vi "SigGenPwrMtr.vi"() -> ()   [LabVIEW 2009]
panel:
  out "Power returned (dBm)":dbl(graph)
  in  "RF Power Level (dBm)":dbl=-80.0 min=-120.0 max=20.0 step=2.0 format="%#_9g"
  in  "RF Frequency  (GHz)":dbl=2.809 min=0.6 max=3.0 step=0.001 format="%#_9g"
  out "RF Power":bool
  in  "RF ON/OFF":bool
  in  "SET FREQ":bool
  in  "SET POWER":bool
  out "Power":dbl
  out "Freq (GHz)":dbl format="%#_10e"
  in  "error in (no error)":errorcluster
  out "error out":errorcluster
  in  "STATUS":bool
  in  "STOP":bool
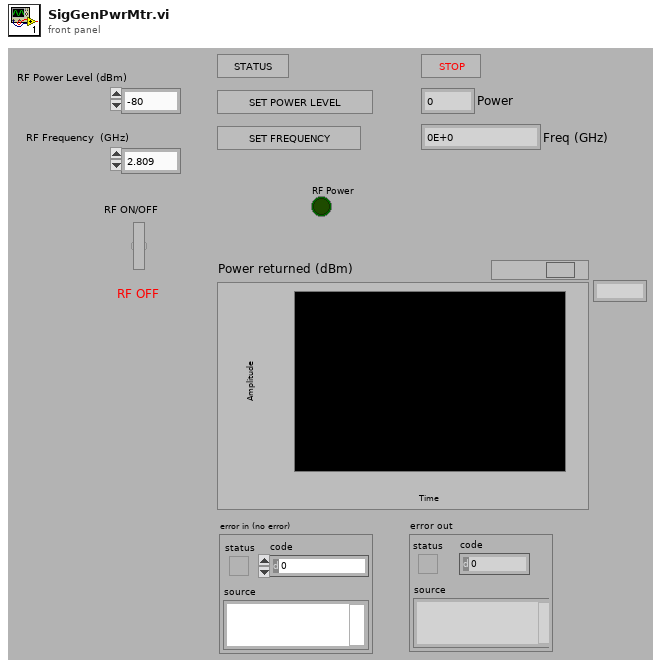
[diagram p1: front panel]
types:
  T1 = enum16{"N1911A", "Siggen", "34980a", "E4418B", "Rvp8"}
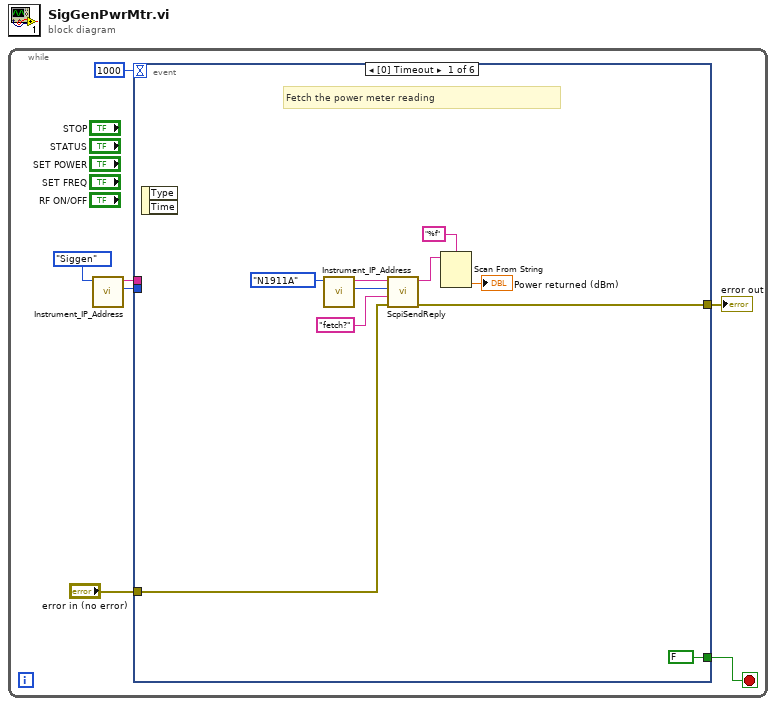
[diagram p0: block diagram]
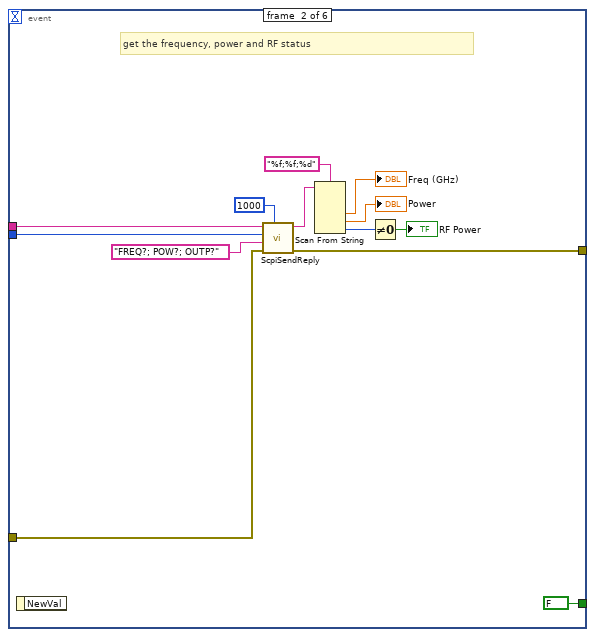
[diagram p2: hidden frame]
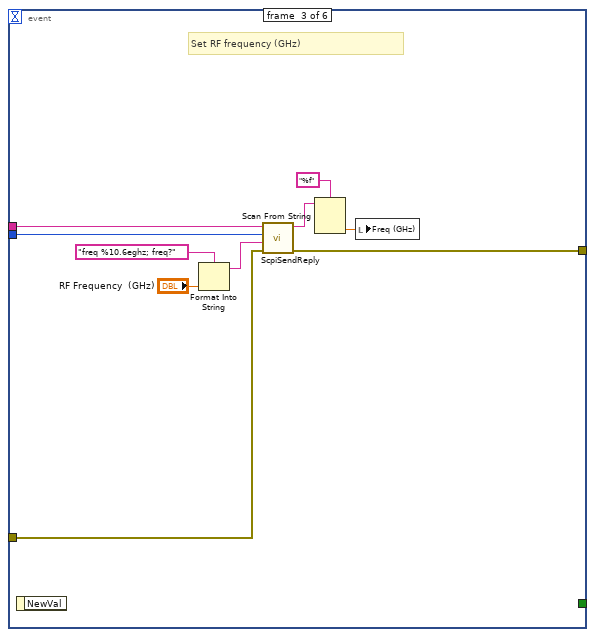
[diagram p3: hidden frame]
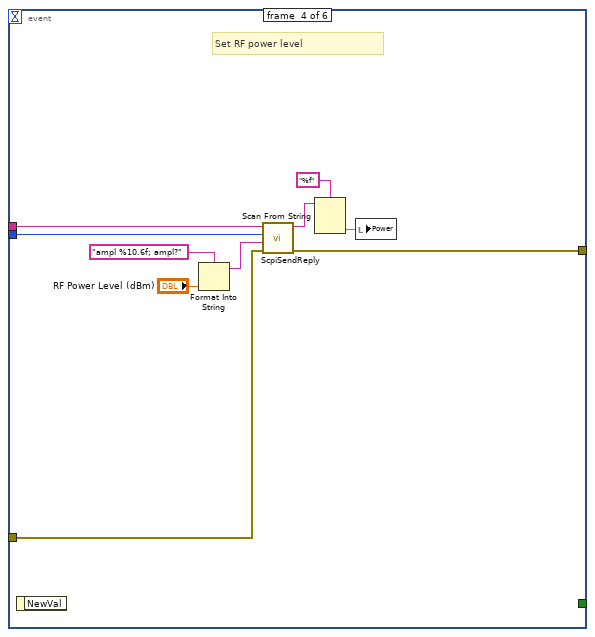
[diagram p4: hidden frame]
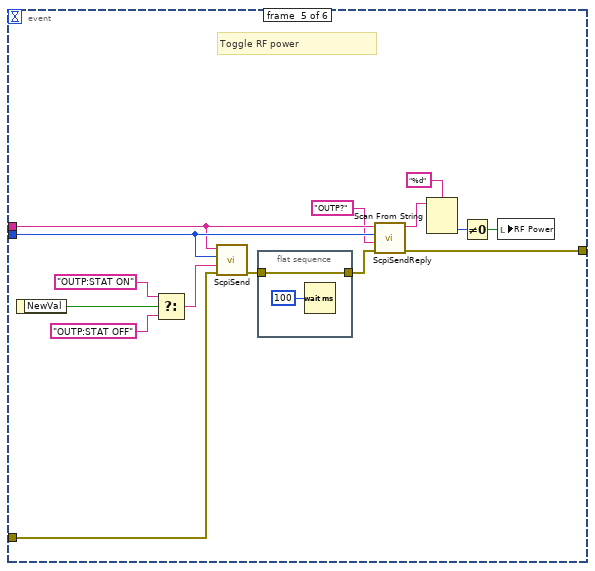
[diagram p5: hidden frame]
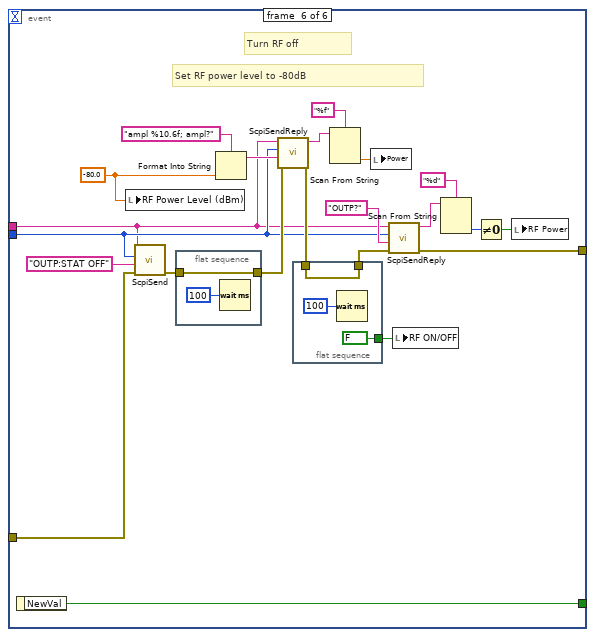
[diagram p6: hidden frame]
diagram:
  n1 = while {
    stop <- w7 stop-if-true
    n2 = call "Instrument_IP_Address.vi"("Instrument"=T1."Siggen") -> ("Port"=w1:u16, "IP Address"=w2:string)  [unwired: 9 in]
    n3 = event shown="[0] Timeout" {
      selector: _ -> [_ _ _ _ _ _]
      dyn-events: _ -> [_ _ _ _ _ _]
      timeout: 1000 -> [_ _ _ _ _ _]
      tunnel: [FALSE ("NewVal") FALSE ("NewVal") _ _ _ w89] -> w7
      tunnel: "error in (no error)" -> [w9 w28 w32 w43 w55 w83]
      tunnel: [w8 w27 w31 w42 w59 w82] -> w5
      tunnel: w2 -> [_ w19 w34 w45 w57 w70]
      tunnel: w1 -> [_ w18 w33 w44 w58 w71]
      event #0 {
        # "Fetch the power meter reading"
        n4 = event-data() -> ()  [unwired: 1 in, 2 out]
        n5 = call "Instrument_IP_Address.vi"("Instrument"=T1."N1911A") -> ("Port"=w16:u16, "IP Address"=w15:string)  [unwired: 9 in]
        n6 = call "ScpiSendReply.vi"("error in (no error)"=w9, "Command"="fetch?" ("format string"), "TCP port"=w16, "IP Address"=w15) -> ("Error out"=w8:errorcluster, "Reply"=w11:string)  [unwired: 5 in]
        n7 = Scan From String(format string="%f", input string=w11) -> (output 1=→"Power returned (dBm)":dbl)  [unwired: 3 in, 3 out]
      }
      event #1 {
        # "get the frequency, power and RF status"
        n8 = event-data() -> ()  [unwired: 1 in, 1 out]
        n9 = call "ScpiSendReply.vi"("TCP Timeout mS"=1000, "error in (no error)"=w28, "Command"="FREQ?; POW?; OUTP?" ("format string"), "TCP port"=w18, "IP Address"=w19) -> ("Error out"=w27:errorcluster, "Reply"=w25:string)  [unwired: 4 in]
        n10 = Scan From String(format string="%f;%f;%d", input string=w25) -> (output 1=→"Freq (GHz)":dbl, output 2=→"Power":dbl, output 3=w20:i32)  [unwired: 5 in, 3 out]
        n11 = Not Equal To 0?(x=w20) -> (x != 0?=→"RF Power":bool)
      }
      event #2 {
        # "Set RF frequency (GHz)"
        n12 = event-data() -> ()  [unwired: 1 in, 1 out]
        n13 = Format Into String(format string="freq %10.6eghz; freq?", "RF Frequency  (GHz)") -> (resulting string=w38:string)  [unwired: 2 in, 1 out]
        n14 = call "ScpiSendReply.vi"("error in (no error)"=w32, "Command"=w38, "TCP port"=w33, "IP Address"=w34) -> ("Error out"=w31:errorcluster, "Reply"=w40:string)  [unwired: 5 in]
        n15 = Scan From String(format string="%f", input string=w40) -> (output 1=w35:dbl)  [unwired: 3 in, 3 out]
        n16 = local write "Freq (GHz)"(w35) -> ()
      }
      event #3 {
        # "Set RF power level"
        n17 = event-data() -> ()  [unwired: 1 in, 1 out]
        n18 = Format Into String(format string="ampl %10.6f; ampl?", "RF Power Level (dBm)") -> (resulting string=w48:string)  [unwired: 2 in, 1 out]
        n19 = call "ScpiSendReply.vi"("error in (no error)"=w43, "Command"=w48, "TCP port"=w44, "IP Address"=w45) -> ("Error out"=w42:errorcluster, "Reply"=w50:string)  [unwired: 5 in]
        n20 = Scan From String(format string="%f", input string=w50) -> (output 1=w41:dbl)  [unwired: 3 in, 3 out]
        n21 = local write "Power"(w41) -> ()
      }
      event #4 {
        # "Toggle RF power"
        n22 = event-data() -> ("NewVal"=w63:bool)  [unwired: 1 in]
        n23 = Select(t="OUTP:STAT ON" ("format string"), s=w63, f="OUTP:STAT OFF" ("format string")) -> (s? t:f=w56:string)
        n24 = call "ScpiSend.vi"("error in (no error)"=w55, "Command"=w56, "TCP port"=w58, "IP Address"=w57) -> ("error out"=w53:errorcluster)  [unwired: 7 in]
        n25 = flat-sequence {
          tunnel: w53 -> [w67]
          tunnel: [w67] -> w52
          frame #0 {
            n26 = Wait (ms)(milliseconds to wait=u32 100) -> ()  [unwired: 1 out]
          }
        }
        n27 = call "ScpiSendReply.vi"("error in (no error)"=w52, "Command"="OUTP?" ("format string"), "TCP port"=w58, "IP Address"=w57) -> ("Error out"=w59:errorcluster, "Reply"=w65:string)  [unwired: 5 in]
        n28 = Scan From String(format string="%d", input string=w65) -> (output 1=w51:i32)  [unwired: 3 in, 3 out]
        n29 = Not Equal To 0?(x=w51) -> (x != 0?=w60:bool)
        n30 = local write "RF Power"(w60) -> ()
      }
      event #5 {
        w68 = -80.0 ("input 1")
        # "Set RF power level to -80dB"
        # "Turn RF off"
        n31 = event-data() -> ("NewVal"=w89:bool)  [unwired: 1 in]
        n32 = local write "RF Power Level (dBm)"(w68) -> ()
        n33 = call "ScpiSend.vi"("error in (no error)"=w83, "Command"="OUTP:STAT OFF" ("format string"), "TCP port"=w71, "IP Address"=w70) -> ("error out"=w87:errorcluster)  [unwired: 7 in]
        n34 = flat-sequence {
          tunnel: w87 -> [w94]
          tunnel: [w94] -> w74
          frame #0 {
            n35 = Wait (ms)(milliseconds to wait=u32 100) -> ()  [unwired: 1 out]
          }
        }
        n36 = Format Into String(format string="ampl %10.6f; ampl?", w68) -> (resulting string=w78:string)  [unwired: 2 in, 1 out]
        n37 = call "ScpiSendReply.vi"("error in (no error)"=w74, "Command"=w78, "TCP port"=w71, "IP Address"=w70) -> ("Error out"=w73:errorcluster, "Reply"=w79:string)  [unwired: 5 in]
        n38 = flat-sequence {
          tunnel: w73 -> [w91]
          tunnel: [w91] -> w72
          tunnel: [FALSE ("RF ON/OFF")] -> w69
          frame #0 {
            n39 = Wait (ms)(milliseconds to wait=u32 100) -> ()  [unwired: 1 out]
          }
        }
        n40 = Scan From String(format string="%f", input string=w79) -> (output 1=w75:dbl)  [unwired: 3 in, 3 out]
        n41 = local write "Power"(w75) -> ()
        n42 = call "ScpiSendReply.vi"("error in (no error)"=w72, "Command"="OUTP?" ("format string"), "TCP port"=w71, "IP Address"=w70) -> ("Error out"=w82:errorcluster, "Reply"=w84:string)  [unwired: 5 in]
        n43 = local write "RF ON/OFF"(w69) -> ()
        n44 = Scan From String(format string="%d", input string=w84) -> (output 1=w88:i32)  [unwired: 3 in, 3 out]
        n45 = Not Equal To 0?(x=w88) -> (x != 0?=w80:bool)
        n46 = local write "RF Power"(w80) -> ()
      }
    }
    "error out" <- w5
  }
